vi "wgs84_to_TM.vi"(8 "y(long)":dbl format="%#_13g", 11 "x(lat)":dbl format="%#_13g") -> (0 "TM경도 Y(E)":dbl format="%#_13g", 3 "TM위도 X(N)":dbl format="%#_13g")   [LabVIEW 2015]
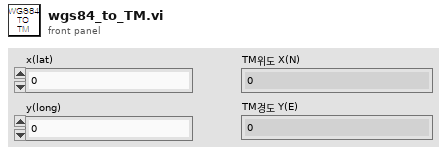
[diagram p1: front panel]
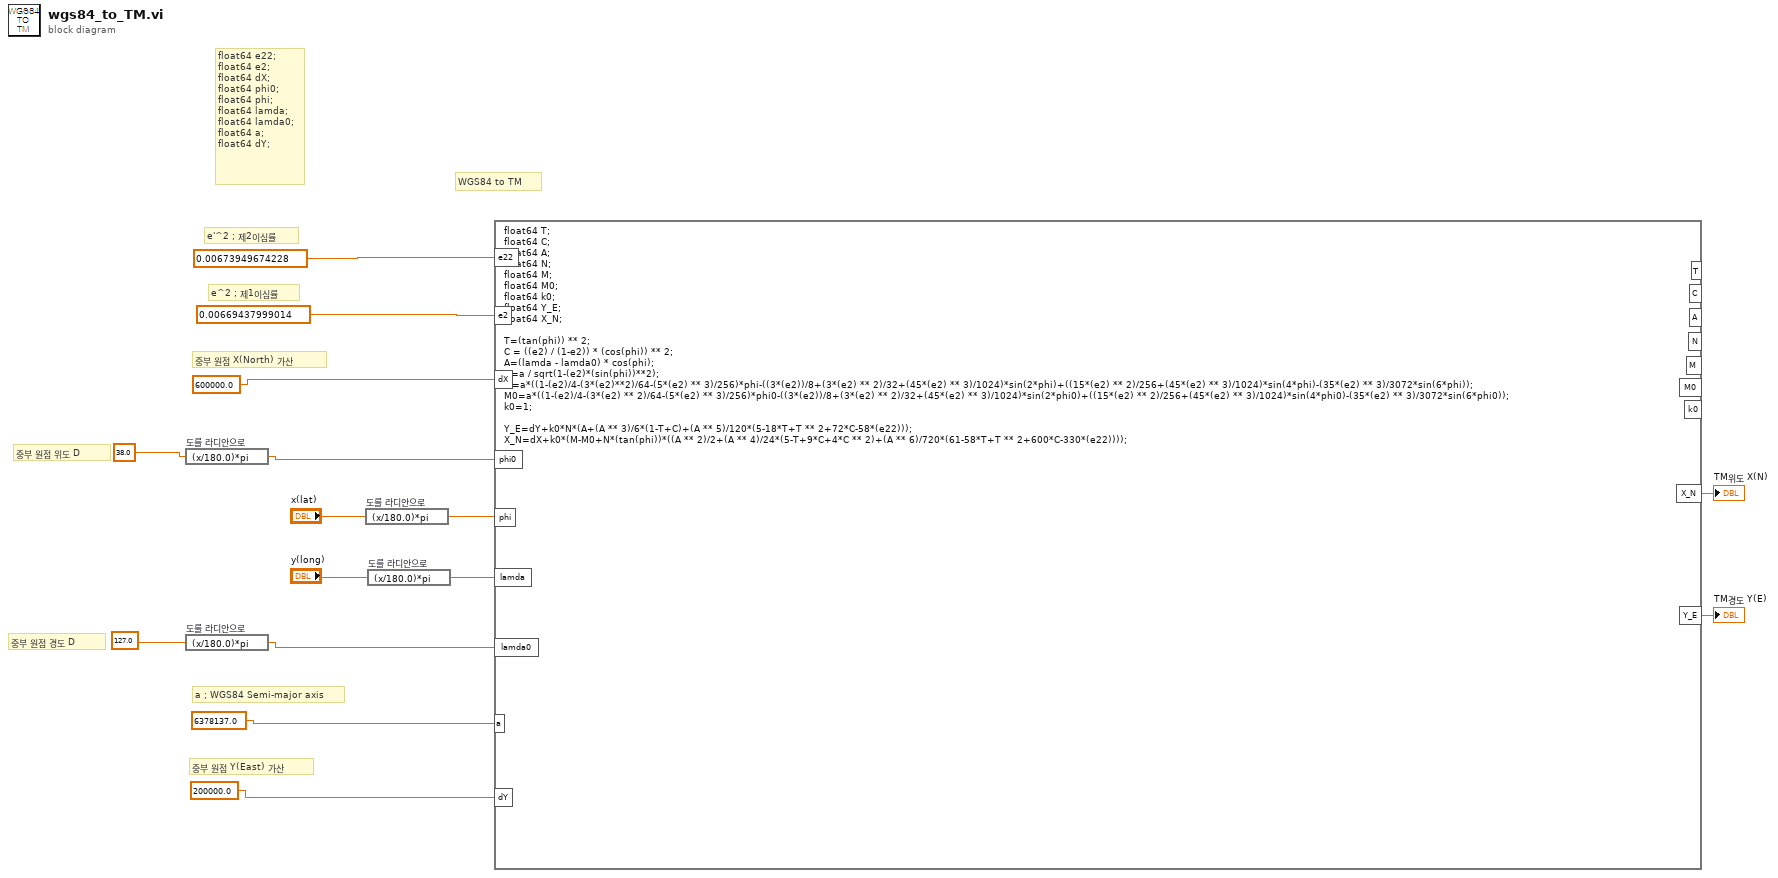
[diagram p0: block diagram]
diagram:
  # "float64 e22;\nfloat64 e2;\nfloat64 dX;\nfloat64 phi0;\nfloat64 phi;\nfloat64 lamda;\nfloat64 lamda0;\nfloat64 a;\nfloat64 dY;"
  # "WGS84 to TM"
  # "a ; WGS84 Semi-major axis"
  # "중부 원점 X(North) 가산"
  # "중부 원점 Y(East) 가산"
  # "e'^2 ; 제2이심률"
  # "중부 원점 경도 D"
  # "중부 원점 위도 D"
  # "e^2 ; 제1이심률"
  n1 = expression code="(x/180.0)*pi" "도를 라디안으로"(38.0) -> (w11:dbl)
  n2 = expression code="(x/180.0)*pi" "도를 라디안으로"(127.0) -> (w10:dbl)
  n3 = expression code="(x/180.0)*pi" "도를 라디안으로"("x(lat)") -> (w6:dbl)
  n4 = expression code="(x/180.0)*pi" "도를 라디안으로"("y(long)") -> (w3:dbl)
  n5 = formula code="float64 T; \nfloat64 C;\nfloat64 A; \nfloat64 N; \nfloat64 M; \nfloat64 M0; \nfloat64 k0; \nfloat64 Y_E; \nfloat64 X_N;\n\nT=(tan(phi)) ** 2;\nC = ((e2) / (1-e2)) * (cos(phi)) ** 2;\nA=(lamda - lamda0) * cos(phi);\nN=a / sqrt(1-(e2)*(sin(phi))**2);\nM=a*((1-(e2)/4-(3*(e2)**2)/64-(5*(e2) ** 3)/256)*phi-((3*(e2))/8+(3*(e2) ** 2)/32+(45*(e2) ** 3)/1024)*sin(2*phi)+((15*(e2) ** 2)/256+(45*(e2) ** 3)/1024)*sin(4*phi)-(35*(e2) ** 3)/3072*sin(6*phi));\nM0=a*((1-(e2)/4-(3*(e2) ** 2)/64-(5*(e2) ** 3)/256)*phi0-((3*(e2))/8+(3*(e2) ** 2)/32+(45*(e2) ** 3)/1024)*sin(2*phi0)+((15*(e2) ** 2)/256+(45*(e2) ** 3)/1024)*sin(4*phi0)-(35*(e2) ** 3)/3072*sin(6*phi0));\nk0=1;\n\nY_E=dY+k0*N*(A+(A ** 3)/6*(1-T+C)+(A ** 5)/120*(5-18*T+T ** 2+72*C-58*(e22)));\nX_N=dX+k0*(M-M0+N*(tan(phi))*((A ** 2)/2+(A ** 4)/24*(5-T+9*C+4*C ** 2)+(A ** 6)/720*(61-58*T+T ** 2+600*C-330*(e22))));"("e2"=0.00669437999014, "dX"=600000.0, "phi0"=w11, "phi"=w6, "lamda"=w3, "lamda0"=w10, "a"=6378137.0, "dY"=200000.0, "e22"=0.00673949674228) -> ("X_N"=→"TM위도 X(N)":dbl, "Y_E"=→"TM경도 Y(E)":dbl)  [unwired: 7 out]
